vi "QDM matlab saver_101freqs_rt_OBD092319.vi"(3 "numOfFreq":enum16{""}(ring), 4 "numFreqs":i32=101, 6 "img data stack Input":dbl[][](array[numeric]), 7 "matlab path":path, 8 "Height":i64(slide)=1200 min=0 max=1200 step=4 scale=0.0..1200.0, 9 "Width":i64(slide)=1920 min=0 max=1920 step=4 scale=0.0..1920.0, 10 "freq list (Hz)":dbl[](array[numeric]), 11 "sweep #":i32) -> ()   [LabVIEW 2018]
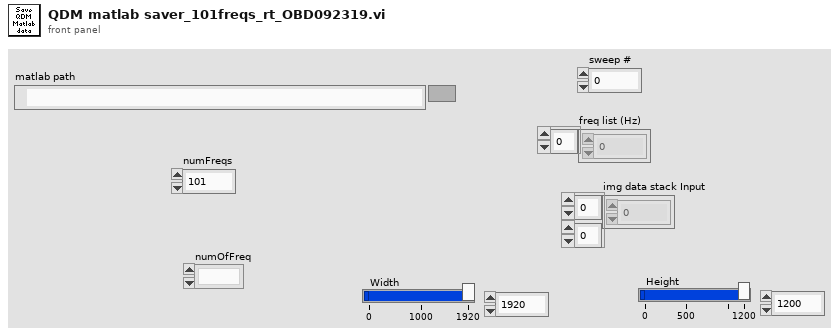
[diagram p1: front panel]
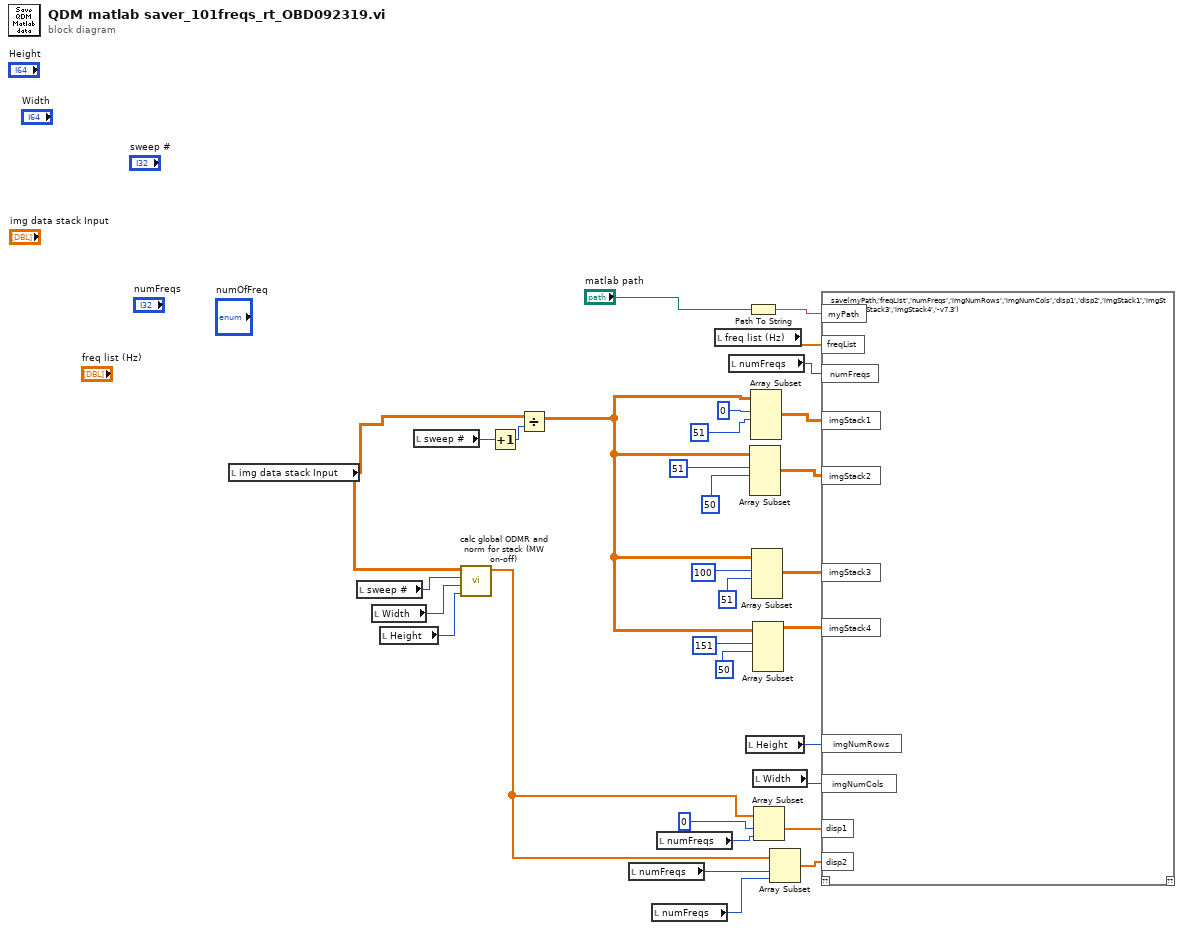
[diagram p0: block diagram]
diagram:
  n1 = local read "img data stack Input"() -> (w11:dbl[][])
  n2 = local read "sweep #"() -> (w12:i32)
  n3 = local read "Width"() -> (w16:i64)
  n4 = local read "Height"() -> (w17:i64)
  n5 = local read "sweep #"() -> (w14:i32)
  n6 = call "calc global ODMR and norm for stack (MW on-off).vi"("Height"=w17, "Width"=w16, "sweep #"=w12, "img data stack"=w11) -> ("normed spectrum"=w15:dbl[])  [unwired: 7 in]
  n7 = Increment(x=w14) -> (x+1=w13:i32)
  n8 = Divide(x=w11, y=w13) -> (x/y=w8:dbl[][])
  n9 = local read "numFreqs"() -> (w25:i32)
  n10 = local read "numFreqs"() -> (w24:i32)
  n11 = local read "numFreqs"() -> (w26:i32)
  n12 = local read "freq list (Hz)"() -> (w31:dbl[])
  n13 = local read "numFreqs"() -> (w30:i32)
  n14 = local read "Height"() -> (w28:i64)
  n15 = Path To String(path="matlab path") -> (string=w32:string)
  n16 = Array Subset(array=w8, index (row)=51, length (row)=50) -> (w18:dbl[][])  [unwired: 2 in]
  n17 = Array Subset(array=w8, index (row)=0 ("index"), length (row)=51) -> (w19:dbl[][])  [unwired: 2 in]
  n18 = Array Subset(array=w8, index (row)=100, length (row)=51) -> (w2:dbl[][])  [unwired: 2 in]
  n19 = Array Subset(array=w8, index (row)=151, length (row)=50) -> (w1:dbl[][])  [unwired: 2 in]
  n20 = local read "Width"() -> (w29:i64)
  n21 = Array Subset(array=w15, index=0, length=w26) -> (w23:dbl[])
  n22 = Array Subset(array=w15, index=w25, length=w24) -> (w22:dbl[])
  n23 = script code="save(myPath,'freqList','numFreqs','imgNumRows','imgNumCols','disp1','disp2','imgStack1','imgStack2','imgStack3','imgStack4','-v7.3')"("myPath"=w32, "freqList"=w31, "imgStack1"=w19, "numFreqs"=w30, "imgNumRows"=w28, "imgNumCols"=w29, "disp1"=w23, "disp2"=w22, "imgStack2"=w18, "imgStack3"=w2, "imgStack4"=w1) -> ()  [unwired: 1 in, 1 out]
